vi "Lumberjack File Test.vi"() -> ()   [LabVIEW 2026]
uses:
  src/TypeDefs/FileAppenderConfig.ctl
  src/TypeDefs/AppenderConfig.ctl
  src/TypeDefs/Severity.ctl
  src/TypeDefs/Filter.ctl
  src/TypeDefs/FilterMode.ctl
  src/TypeDefs/DropPolicy.ctl
  src/TypeDefs/FileConfig.ctl
  src/Public/Logger.lvclass/Logger.lvclass
  src/Lumberjack.lvlib
panel:
  in  "Enable Default File":bool=TRUE
  in  "Host Application":path=path "C:/Users/dallis/OneDrive - Velico Medical/Documents/Personal/LabVIEW Coding Projects/Lumberjack"
  in  "File Appender Configuration":T1={"common"={"id"="default", "threshold"=enum."ALL", "filter"={"mode"=enum."Mirror", "levelMin"=enum."ALL", "levelMax"=enum."ALL", "tagPrefix"=""}, "queueBound"=-1, "dropPolicy"=enum."DropOldest", "useUTC"=TRUE}, "file"={"rootFolder"=path "C:/Users/dallis/OneDrive - Velico Medical/Desktop/Test", "maxFileSize"=10485760, "maxFileCount"=1, "baseName"="smoketest", "extension"="CSV", "delimiter"=",", "calendarFolderTree"=FALSE}}
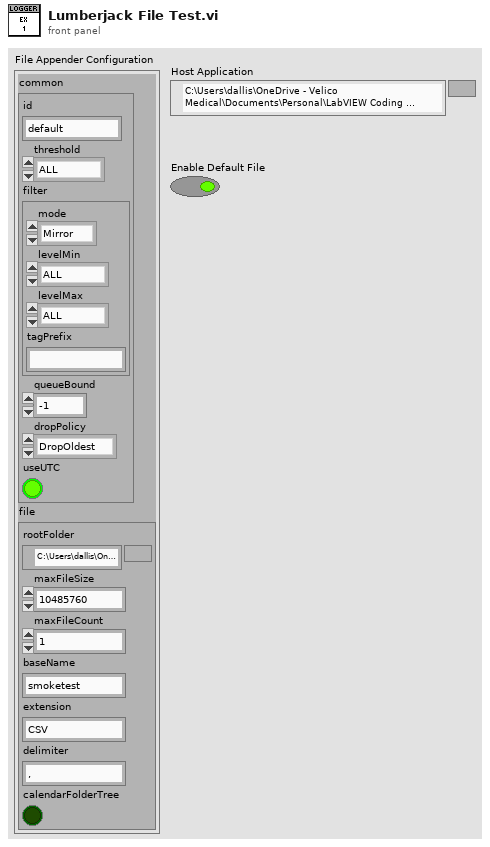
[diagram p1: front panel]
types:
  T1 = typedef "Lumberjack.lvlib/FileAppenderConfig.ctl" = cluster{"common":T2, "file":T7}
  T2 = typedef "Lumberjack.lvlib/AppenderConfig.ctl" = cluster{"id":string, "threshold":T3, "filter":T4, "queueBound":i32, "dropPolicy":T6, "useUTC":bool}
  T3 = typedef "Lumberjack.lvlib/Severity.ctl" = enum16{"OFF", "FATAL", "ERROR", "WARN", "INFO", "DEBUG", "TRACE", "ALL"}
  T4 = typedef "Lumberjack.lvlib/Filter.ctl" = cluster{"mode":T5, "levelMin":T3, "levelMax":T3, "tagPrefix":string}
  T5 = typedef "Lumberjack.lvlib/FilterMode.ctl" = enum16{"Mirror", "Routed"}
  T6 = typedef "Lumberjack.lvlib/DropPolicy.ctl" = enum16{"DropOldest", "DropNewest", "LevelAware"}
  T7 = typedef "Lumberjack.lvlib/FileConfig.ctl" = cluster{"rootFolder":path, "maxFileSize":i64, "maxFileCount":i32, "baseName":string, "extension":string, "delimiter":string, "calendarFolderTree":bool}
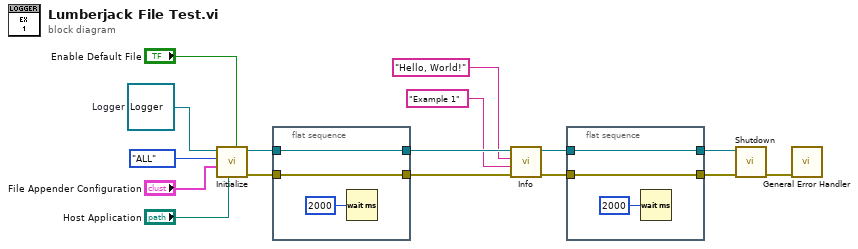
[diagram p0: block diagram]
diagram:
  w6 = refnum<class "Logger.lvclass"> refnum  # Logger
  n1 = call "Initialize.vi"("enableDefaultFile"="Enable Default File", "hostApplicationPath"="Host Application", "defaultFileAppender"="File Appender Configuration", "initialGlobalThreshold"=Severity."ALL", "Logger in"=w6) -> ("error out"=w14:errorcluster, "Logger out"=w12:refnum<class "Logger.lvclass">)  [unwired: 5 in]
  n2 = flat-sequence {
    tunnel: [w18] -> w13
    tunnel: w14 -> [w18]
    tunnel: w12 -> [w17]
    tunnel: [w17] -> w11
    frame #0 {
      n3 = Wait (ms)(milliseconds to wait=u32 2000) -> ()  [unwired: 1 out]
    }
  }
  n4 = call "Info.vi"("error in (no error)"=w13, "sourceTag"="Example 1", "message"="Hello, World!", "Logger in"=w11) -> ("error out"=w4:errorcluster, "Logger out"=w5:refnum<class "Logger.lvclass">)  [unwired: 6 in]
  n5 = flat-sequence {
    tunnel: [w21] -> w2
    tunnel: w4 -> [w21]
    tunnel: w5 -> [w20]
    tunnel: [w20] -> w3
    frame #0 {
      n6 = Wait (ms)(milliseconds to wait=u32 2000) -> ()  [unwired: 1 out]
    }
  }
  n7 = call "Shutdown.vi"("error in (no error)"=w2, "Logger in"=w3) -> ("error out"=w1:errorcluster)  [unwired: 9 in]
  n8 = call <vilib>:"General Error Handler.vi"("error in (no error)"=w1) -> ()  [unwired: 10 in, 5 out]
